vi "nearest_multiple.vi"(8 "numChan":i32, 11 "N":i32) -> (0 "(int) y*floor(x/y)":u64)   [LabVIEW 2015]
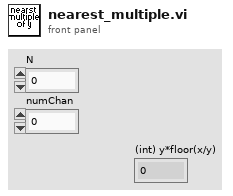
[diagram p1: front panel]
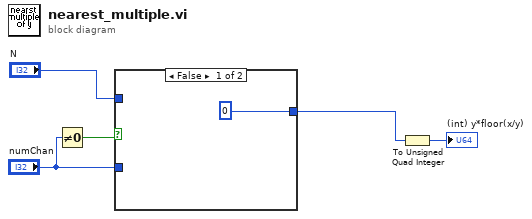
[diagram p0: block diagram]
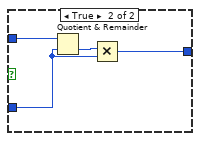
[diagram p2: hidden frame]
diagram:
  n1 = Not Equal To 0?(x="numChan") -> (x != 0?=w2:bool)
  n2 = case shown="False" w2 {
    tunnel: "N" -> [_ w10]
    tunnel: "numChan" -> [_ w8]
    tunnel: [0 w7] -> w4
    frame False {
    }
    frame True {
      n3 = Quotient & Remainder(x=w10, y=w8) -> (floor(x/y)=w9:i32)  [unwired: 1 out]
      n4 = Multiply(x=w9, y=w8) -> (x*y=w7:i32)
    }
  }
  n5 = To Unsigned Quad Integer(1:w4) -> (0:→"(int) y*floor(x/y)":u64)
